vi "SetDistanceFromWall.vi"(7 "Timeout":dbl, 8 "Error In":errorcluster, 9 "Initation?":bool, 10 "MaxSpeed":dbl, 11 "Distance":dbl) -> (0 "Error Out":errorcluster, 2 "Succesful":bool, 3 "Finished":bool)   [LabVIEW 2020]
uses:
  <vilib>/Utility/semaphor.llb/Obtain Semaphore Reference.vi
  <vilib>/Rock Robotics/WPI/ThirdParty/JAS_Junk/TrajLib/Timer_Reset.vi
  DriveGlobals.vi
  <vilib>/Rock Robotics/WPI/ThirdParty/JAS_Junk/TrajLib/Trajectory_Library.lvlib
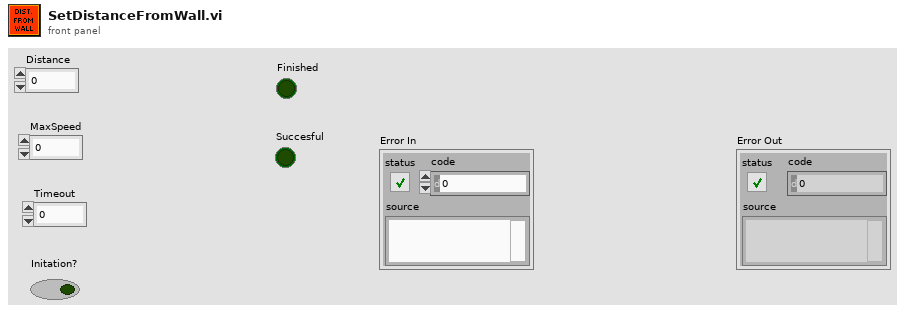
[diagram p1: front panel]
types:
  T1 = typedef "Trajectory_Library.lvlib/TIMER.ctl" = cluster{"StartTime":dbl, "Accumulated TIme":dbl, "Running":bool, "semaphore":T2}
  T2 = typedef "Semaphore RefNum" = refnum<k1>
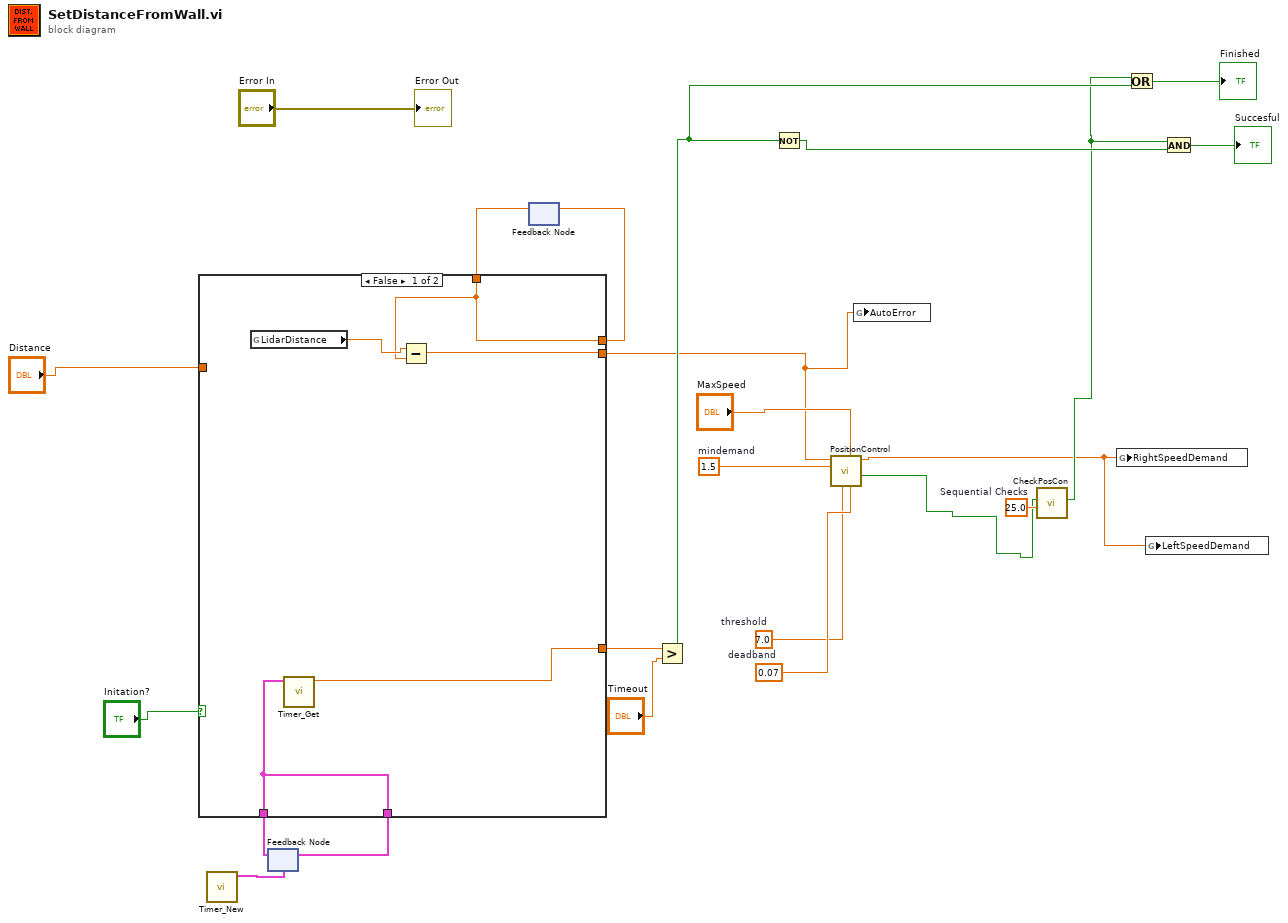
[diagram p0: block diagram]
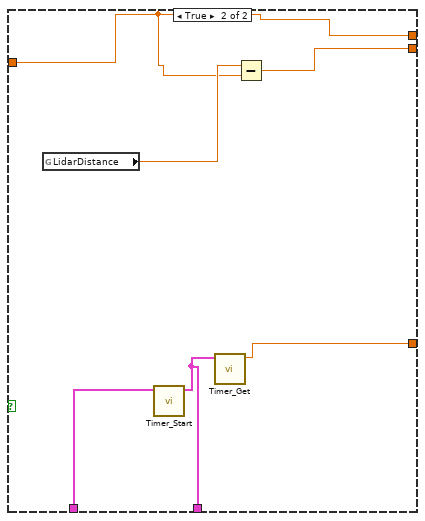
[diagram p2: hidden frame]
diagram:
  w3 = 25.0  # Sequential Checks
  w12 = 0.07  # deadband
  w11 = 7.0  # threshold
  w10 = 1.5  # mindemand
  n1 = call <vilib>:"Timer_New.vi"() -> ("TIMER"=w9:T1)  [unwired: 11 in]
  n2 = feedback #1(w9) -> (w21:T1)
  n3 = feedback #2() -> (w17:dbl)  [unwired: 1 in]
  n4 = case shown="False" "Initation?" {
    tunnel: w21 -> [w26 w33]
    tunnel: "Distance" -> [_ w29]
    tunnel: w17 -> [w24 _]
    tunnel: [w24 w29] -> w18
    tunnel: [w28 w34] -> w13
    tunnel: [w27 w31] -> w5
    tunnel: [w26 w32] -> w8
    frame False {
      n5 = global read "DriveGlobals.vi" "LidarDistance"() -> (w25:dbl)
      n6 = call <vilib>:"Timer_Get.vi"("TIMER"=w26) -> ("CurrentTImer"=w28:dbl)  [unwired: 10 in]
      n7 = Subtract(x=w25, y=w24) -> (x-y=w27:dbl)
    }
    frame True {
      n8 = global read "DriveGlobals.vi" "LidarDistance"() -> (w30:dbl)
      n9 = call <vilib>:"Timer_Start.vi"("in Timer"=w33) -> ("out Timer"=w32:T1)  [unwired: 10 in]
      n10 = call <vilib>:"Timer_Get.vi"("TIMER"=w32) -> ("CurrentTImer"=w34:dbl)  [unwired: 10 in]
      n11 = Subtract(x=w30, y=w29) -> (x-y=w31:dbl)
    }
  }
  n12 = feedback-in #1(w8) -> ()
  n13 = feedback-in #2(w18) -> ()
  n14 = Greater?(x=w13, y="Timeout") -> (0:w6:bool)
  n15 = Not(x=w6) -> (.not. x?=w15:bool)
  n16 = call "PositionControl.vi"("deadband"=w12, "maxdemand"="MaxSpeed", "threshold"=w11, "mindemand"=w10, "Error"=w5) -> ("on target"=w1:bool, "output variable"=w2:dbl)  [unwired: 5 in]
  n17 = global write "DriveGlobals.vi" "AutoError"(w5) -> ()
  n18 = call "CheckPosCon.vi"("Sequential Checks"=w3, "WasRight"=w1) -> ("We made It"=w4:bool)  [unwired: 9 in]
  n19 = global write "DriveGlobals.vi" "RightSpeedDemand"(w2) -> ()
  n20 = Or(x=w4, y=w6) -> (x .or. y?=→"Finished":bool)
  n21 = global write "DriveGlobals.vi" "LeftSpeedDemand"(w2) -> ()
  n22 = And(x=w4, y=w15) -> (x .and. y?=→"Succesful":bool)
  "Error Out" <- "Error In"
